vi "Ratchet.vi"   [LabVIEW 2012]
uses:
  Robot Global Data.vi
  <vilib>/Rock Robotics/WPI/Solenoid/WPI_SolenoidSetEnum.vi
  <vilib>/Rock Robotics/WPI/Solenoid/WPI_SolenoidValue.ctl
types:
  T1 = typedef "WPI_SolenoidDevRef.ctl" = cluster{"DevStatus":errorcluster, "Solenoid Module":T2, "Forward Solenoid Channel":T3, "Reverse Solenoid Channel":T3}
  T2 = typedef "FPGA_TypedefSolenoidModule.ctl" = enum16{"Solenoid Module 1", "Solenoid Module 2"}
  T3 = typedef "WPI_SolenoidChannel.ctl" = enum8{"Solenoid 1", "Solenoid 2", "Solenoid 3", "Solenoid 4", "Solenoid 5", "Solenoid 6", "Solenoid 7", "Solenoid 8", "Invalid"}
  T4 = typedef "WPI_SolenoidValue.ctl" = enum16{"Off", "On", "Forward", "Reverse"}
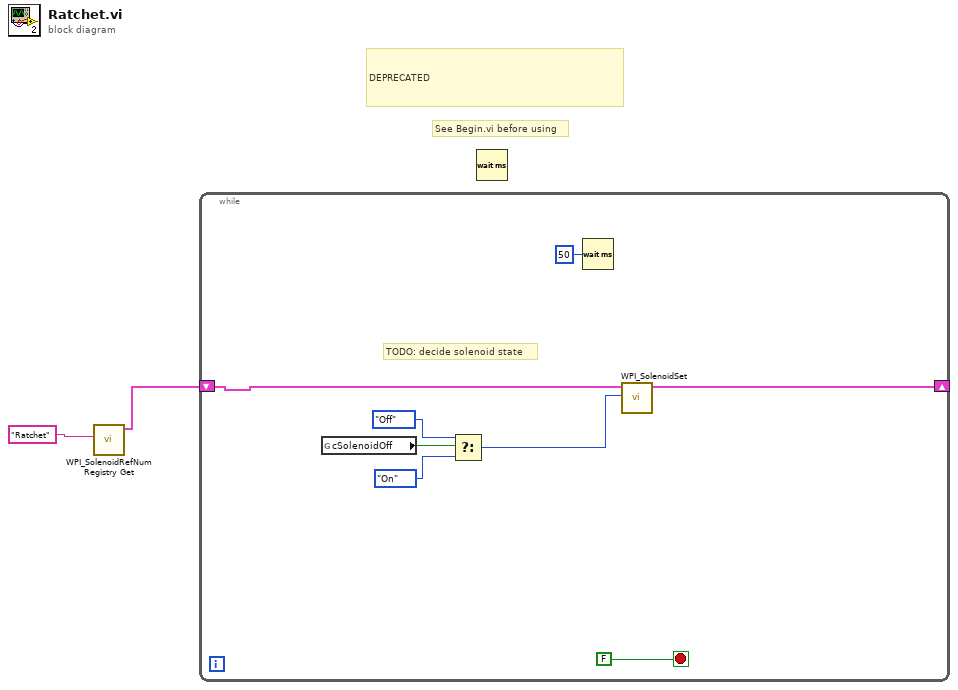
[diagram p0: block diagram]
diagram:
  # "See Begin.vi before using"
  # "DEPRECATED"
  n1 = call <vilib>:"WPI_SolenoidRefNum Registry Get.vi"("refnum name"="Ratchet") -> ("SolenoidDevRef"=w1:T1)  [unwired: 9 in, 1 out]
  n2 = while {
    shift-right: [w7] -> _
    shift-left: w1 -> [w9]
    stop <- FALSE stop-if-true
    # "TODO: decide solenoid state"
    n3 = global read "Robot Global Data.vi" "cSolenoidOff"() -> (w6:bool)
    n4 = Select(t=WPI_SolenoidValue."Off" ("Value"), s=w6, f=WPI_SolenoidValue."On" ("Value")) -> (s? t:f=w3:T4)
    n5 = Wait (ms)(milliseconds to wait=u32 50) -> ()  [unwired: 1 out]
    n6 = call-poly <vilib>:"WPI_SolenoidSet.vi"("Value"=w3, "SolenoidDevRef"=w9) -> ("SolenoidDevRef"=w7:T1)  [unwired: 8 in, 1 out]
  }
  n7 = Wait (ms)() -> ()  [unwired: 1 in, 1 out]
